vi "Assert To Report Entry.vi"(8 "error in (no error)":errorcluster, 10 "Assert Event Data":T1={"name"="", "passed"=FALSE, "call-chain"=[], "test-error"={"status"=FALSE, "code"=0, "source"=""}, "timestamp"=timestamp(0 s since 1904-01-01), "assert-id"="", "test-id"="", "time"=-1.0, "message"="", "properties"=variant, "measurements"=variant, "user-defined"=variant}) -> (0 "error out":errorcluster, 2 "String":string)   [LabVIEW 2020, in "Caraya.lvlib" / "Test Report.Template.lvclass"]
uses:
  Test Report.Template.lvclass
  Test Result/Assert Event Data (Extended).ctl
  Test Report/Test Report.lvclass
  Test Result/Test Result.lvclass
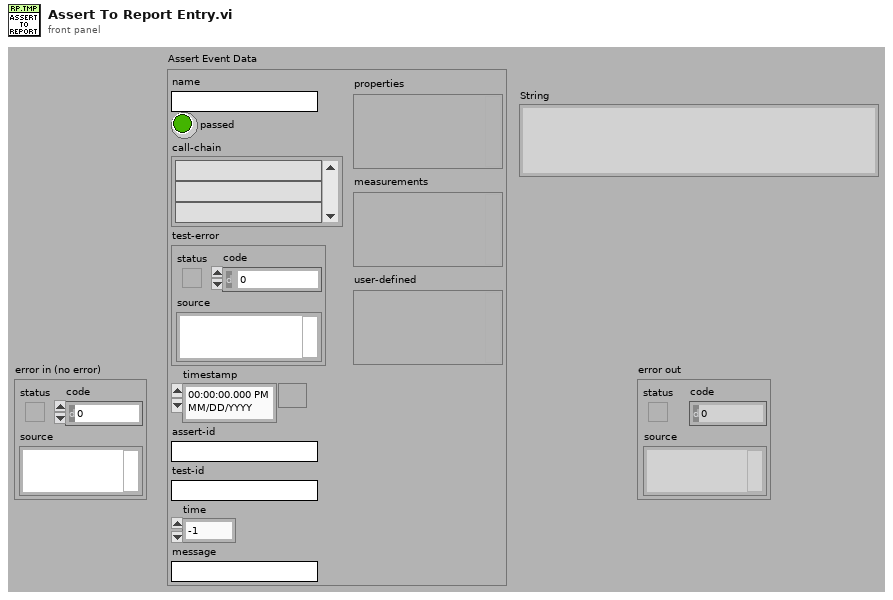
[diagram p1: front panel]
types:
  T1 = typedef "Caraya.lvlib/Test Result.lvclass/Assert Event Data (Extended).ctl" = cluster{"name":string, "passed":bool, "call-chain":string[], "test-error":errorcluster, "timestamp":timestamp, "assert-id":string, "test-id":string, "time":dbl, "message":string, "properties":variant, "measurements":variant, "user-defined":variant}
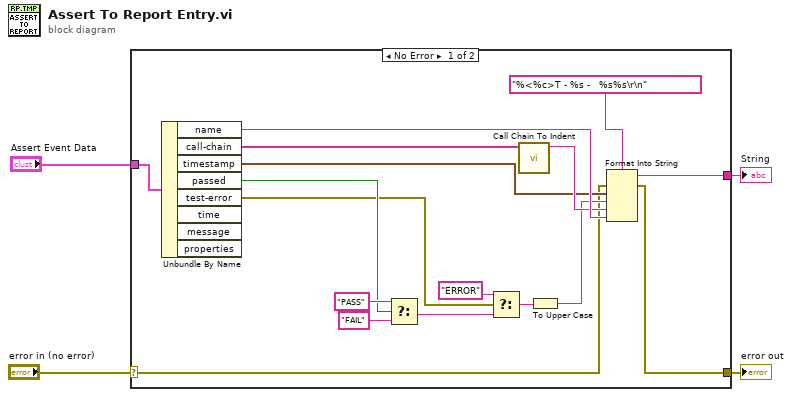
[diagram p0: block diagram]
diagram:
  n1 = case shown="No Error" "error in (no error)" {
    selector: "error in (no error)" -> [w9 w22]
    tunnel: [w19 w22] -> w3
    tunnel: "Assert Event Data" -> [w16 _]
    tunnel: [w18 _] -> w1
    frame No Error {
      n2 = Unbundle By Name(w16) -> ("name"=w20:string, "call-chain"=w15:string[], "timestamp"=w14:timestamp, "passed"=w6:bool, "test-error"=w5:errorcluster)  [unwired: 3 out]
      n3 = Select(t="PASS" ("format string"), s=w6, f="FAIL" ("format string")) -> (s? t:f=w8:string)
      n4 = Select(t="ERROR" ("format string"), s=w5, f=w8) -> (s? t:f=w11:string)
      n5 = call "Call Chain To Indent.vi"("Call Chain"=w15) -> ("Indent"=w17:string)  [unwired: 10 in]
      n6 = To Upper Case(1:w11) -> (0:w10:string)
      n7 = Format Into String(format string="%<%c>T - %s -   %s%s\r\n", error in=w9, w14, w10, w17, w20) -> (resulting string=w18:string, error out=w19:errorcluster)  [unwired: 1 in]
    }
    frame Error {
    }
  }
  "error out" <- w3
  "String" <- w1
